vi "QuadRotor_Monitoring_WithGoogleMap.vi"() -> ()   [LabVIEW 2015]
uses:
  <vilib>/Instr/_visa.llb/VISA Set IO Buffer Mask.ctl
  <vilib>/Instr/_visa.llb/VISA Configure Serial Port (Instr).vi
panel:
  in  "Lontitude_Home":dbl=100.110974 format="%#.6g"
  in  "Latitude_Home":dbl=20.029151 format="%#.6g"
  out "URL":string="http://maps.google.com/staticmap?center=51.406200,-1.307000&zoom=18&size=570x350&maptype=hybrid&markers=51.406200,-1.307000,midpurplea&key=&path=rgb:0xFF1000,weight:5|51.406200,-1.307000|51.406200,-1.307000"
  in  "Zoom":sgl=17.0 format="%#.1g"
  in  "Y":dbl=1000.0
  in  "X":dbl=350.0
  in  "Map Format":string(combo)="hybrid"
  in  "color":string(combo)="orange"
  in  "character":string="Q"
  in  "Path Collor":u32(colorbox)=16715776
  in  "Weight":i32=5
  in  "Show Path?":bool=TRUE
  in  "Home Char":string="H"
  in  "Color":string(combo)="blue"
  in  "?":refnum<k7>(container)
  out "Target_LON":ext format="%#.7f"
  out "Target_LAT":ext format="%#.7f"
  in  "Lontitude_W3":i32=1005738310
  in  "Latitude_W3":i32=139458720
  in  "Lontitude_W2":i32=1005738310
  in  "Latitude_W2":i32=139458720
  in  "Lontitude_W1":i32=1005738310
  in  "Latitude_W1":i32=139458720
  in  "Lon_home":i32=1005748870
  in  "Lat_home":i32=139456050
  out "(GPS_numSat)":u16
  out "return count 2":u32
  out "Roob":i32
  out "Altitude_(Auto)":ext format="%#_3g"
  in  "Set_Altitude_(Auto)":dbl=2.5
  out "string":string
  out "Mode":ext format="%.2f"
  out "Altitude":dbl(slide) scale=0.0..20.0
  out "Altitude":ext format="%.2f"
  out "Yaw":dbl(knob) scale=-180.0..180.0
  out "Pitch":dbl(knob) scale=-90.0..90.0
  out "Roll":dbl(knob) scale=-90.0..90.0
  in  "Write to Quad":bool
  out "Header_58":u8
  out "GPS_Longtitude":ext format="%#.7f"
  out "Pitch":ext format="%.2f"
  out "Yaw":ext format="%.2f"
  out "GPS_Latitude":ext format="%#.7f"
  out "Roll":ext format="%.2f"
  out "return count":u32
  in  "stop":bool
  in  "VISA Serial Data":refnum<visa-resource-name>
  # "Development Autonomous Quad-Rotor Flight Controller for Medical Delivery"
  # "Home Position"
  # "9 Point"
  # "10 Point"
  # "QuadRotor Position"
  # "Data Write to Autonomous Quad Rotor (LAT 9 Point), (LON 10 Point)"
  # "Ex  13.8591411 = 138591411 , 100.5231704 = 1005231704 Using in integer  I32"
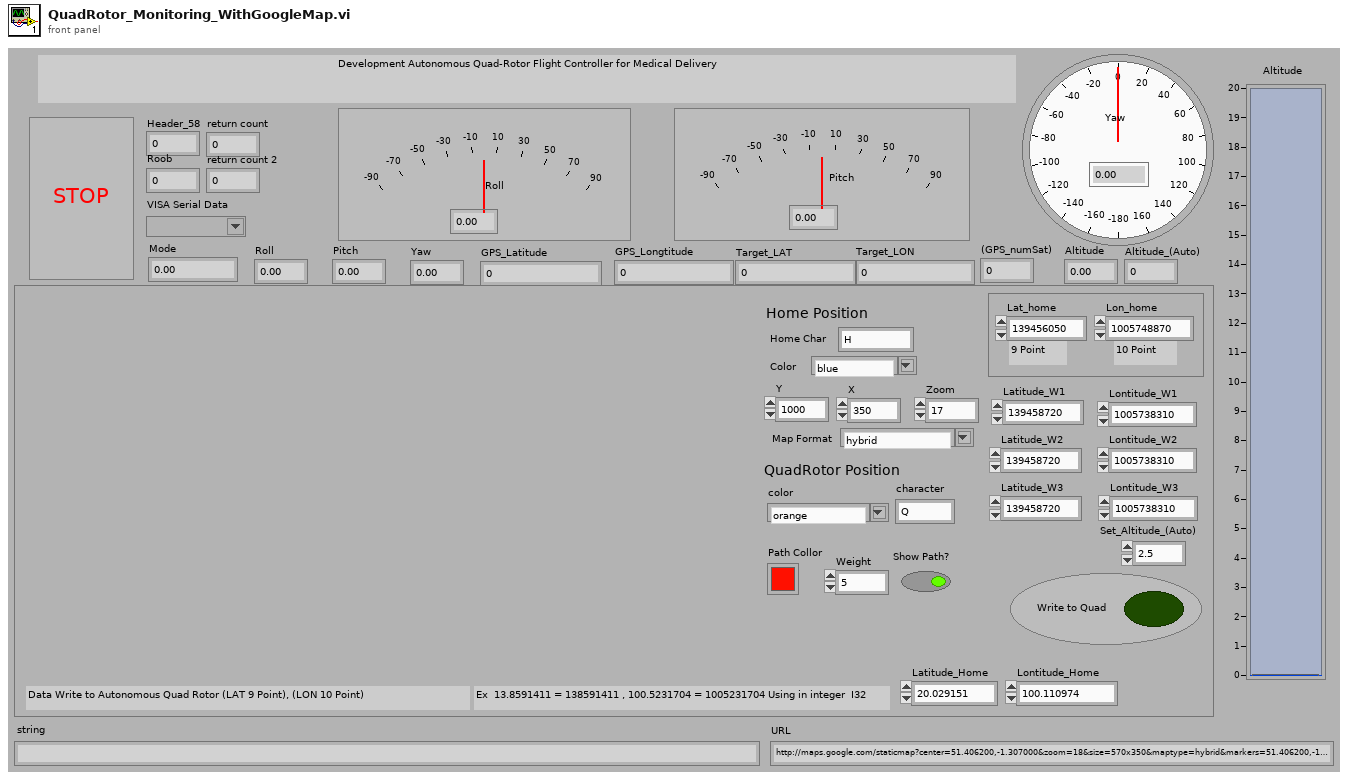
[diagram p1: front panel]
types:
  T1 = typedef "VISA Set IO Buffer Mask.ctl" = u16
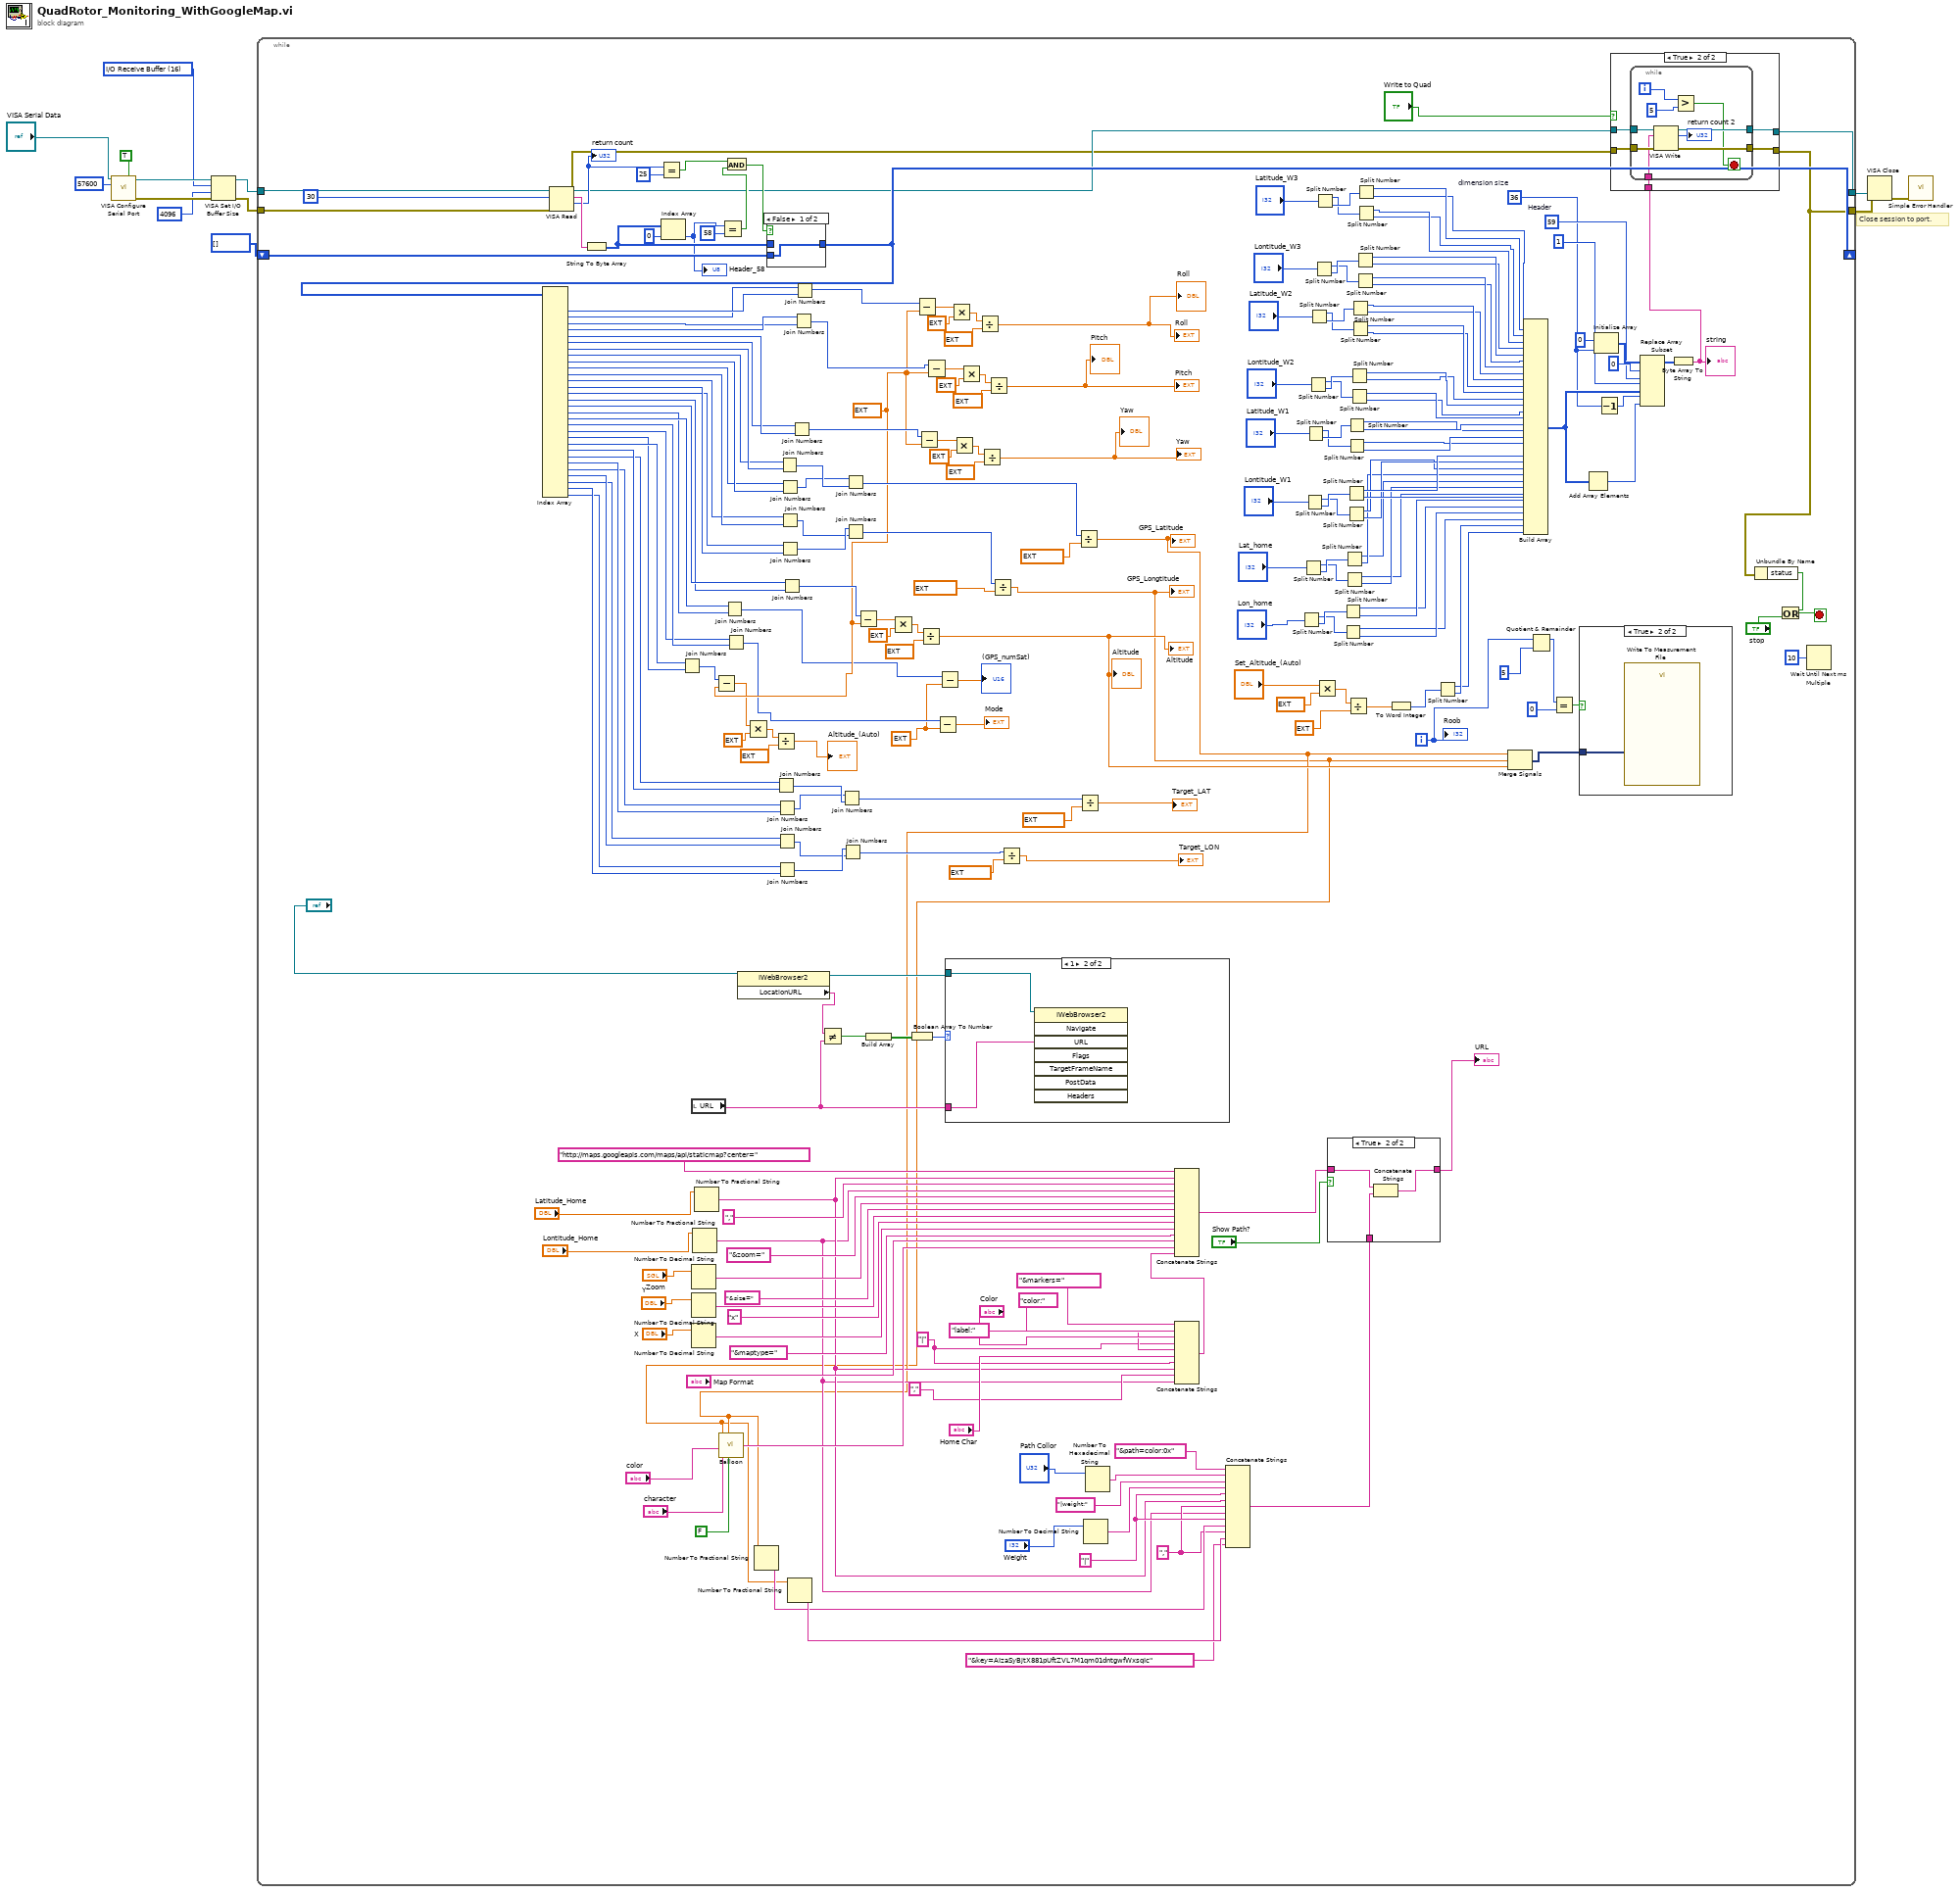
[diagram p0: block diagram]
diagram:
  w10 = T1 16 items=["I/O Receive Buffer"=16, "I/O Transmit Buffer"=32, "I/O Receive and Transmit Buffer"=48] ("Mask")
  # "Close session to port."
  n1 = call-poly "VISA Configure Serial Port"("VISA resource name"="VISA Serial Data", "Enable Termination\nChar (T)"=TRUE ("Enable Termination\nChar (T)"), "baud rate (9600)"=u32 57600) -> ("VISA resource name out"=w12:refnum<visa-resource-name>, "error out"=w11:errorcluster)  [unwired: 7 in, 4 out]
  n2 = VISA Set I/O Buffer Size(VISA resource name=w12, mask (16)=w10, size (4096)=u32 4096, error in (no error)=w11) -> (VISA resource name out=w8:refnum<visa-resource-name>, error out=w6:errorcluster)
  n3 = while {
    tunnel: [w211] -> w7
    tunnel: w8 -> [w252]
    tunnel: [w210] -> w5
    tunnel: w6 -> [w251]
    shift-right: [w221] -> _
    shift-left: u8[] [] ("unsigned byte array") -> [w222]
    i -> [w71]
    stop <- w255 stop-if-true
    w24 = "|"
    w30 = "," ("string")
    w31 = "|"
    w129 = 36  # dimension size
    w178 = u8 59  # Header
    w123 = ext 255.0 ("y")
    w139 = ext 32767.0 ("y")
    n4 = VISA Read(VISA resource name=w252, byte count=u32 30, error in (no error)=w251) -> (VISA resource name out=w213:refnum<visa-resource-name>, read buffer=w225:string, return count=w218:u32, error out=w212:errorcluster)
    "return count" <- w218
    n5 = String To Byte Array(string=w225) -> (unsigned byte array=w223:u8[])
    n6 = Equal?(x=w218, y=u32 25) -> (x = y?=w216:bool)
    n7 = Index Array(array=w223, index=0) -> (element=w215:u8)
    "Header_58" <- w215
    n8 = local read "URL"() -> (w60:string)
    n9 = Number To Decimal String(number="Zoom") -> (decimal integer string=w55:string)  [unwired: 1 in]
    n10 = Number To Decimal String(number="Y") -> (decimal integer string=w51:string)  [unwired: 1 in]
    n11 = Number To Decimal String(number="X") -> (decimal integer string=w49:string)  [unwired: 1 in]
    n12 = Number To Fractional String(number="Lontitude_Home") -> (F-format string=w21:string)  [unwired: 3 in]
    n13 = Number To Fractional String(number="Latitude_Home") -> (F-format string=w22:string)  [unwired: 3 in]
    n14 = Equal?(x=w215, y=u8 58) -> (x = y?=w220:bool)
    n15 = And(x=w216, y=w220) -> (x .and. y?=w219:bool)
    n16 = property class="IWebBrowser2"(reference="?") -> (reference out=w65:refnum<k7>, "LocationURL"=w63:string)  [unwired: 1 in, 1 out]
    n17 = case shown="False" w219 {
      tunnel: w223 -> [_ w280]
      tunnel: [w279 w280] -> w221
      tunnel: w222 -> [w279 _]
      frame False {
      }
      frame True {
      }
    }
    n18 = Index Array(array=w221) -> (element #2=w245:u8, element #3=w244:u8, element #4=w242:u8, element #5=w243:u8, element #6=w249:u8, element #7=w248:u8, element #8=w247:u8, element #9=w246:u8, element #10=w206:u8, element #11=w205:u8, element #12=w202:u8, element #13=w201:u8, element #14=w200:u8, element #15=w199:u8, element #16=w189:u8, element #17=w195:u8, element #18=w187:u8, element #19=w188:u8, element #20=w186:u8, element #21=w185:u8, element #22=w141:u8, element #23=w142:u8, element #24=w79:u8, element #25=w78:u8, element #26=w77:u8, element #27=w76:u8, element #28=w75:u8, element #29=w74:u8, element #30=w73:u8, element #31=w72:u8)  [unwired: 31 in, 1 out]
    n19 = Join Numbers(hi=w142, lo=w141) -> ((hi.lo)=w140:u16)
    n20 = Subtract(x=w140, y=w139) -> (x-y=w135:ext)
    n21 = Join Numbers(hi=w188, lo=w187) -> ((hi.lo)=w122:u16)
    n22 = Join Numbers(hi=w185, lo=w186) -> ((hi.lo)=w126:u16)
    n23 = Multiply(x=w135, y=ext 100.0) -> (x*y=w137:ext)
    n24 = Divide(x=w137, y=ext 32767.0) -> (x/y=→"Altitude_(Auto)":ext)
    n25 = Join Numbers(hi=w78, lo=w79) -> ((hi.lo)=w82:u16)
    n26 = Join Numbers(hi=w76, lo=w77) -> ((hi.lo)=w81:u16)
    n27 = Join Numbers(hi=w74, lo=w75) -> ((hi.lo)=w83:u16)
    n28 = Join Numbers(hi=w72, lo=w73) -> ((hi.lo)=w84:u16)
    n29 = Join Numbers(hi=w246, lo=w247) -> ((hi.lo)=w204:u16)
    n30 = Join Numbers(hi=w205, lo=w206) -> ((hi.lo)=w203:u16)
    n31 = Join Numbers(hi=w201, lo=w202) -> ((hi.lo)=w183:u16)
    n32 = Join Numbers(hi=w199, lo=w200) -> ((hi.lo)=w184:u16)
    n33 = Join Numbers(hi=w195, lo=w189) -> ((hi.lo)=w190:u16)
    n34 = Join Numbers(hi=w248, lo=w249) -> ((hi.lo)=w231:u16)
    n35 = Join Numbers(hi=w243, lo=w242) -> ((hi.lo)=w226:u16)
    n36 = Join Numbers(hi=w244, lo=w245) -> ((hi.lo)=w240:u16)
    n37 = Not Equal?(x=w63, y=w60) -> (x != y?=w64:bool)
    n38 = Join Numbers(hi=w81, lo=w82) -> ((hi.lo)=w80:u32)
    n39 = Join Numbers(hi=w84, lo=w83) -> ((hi.lo)=w86:u32)
    n40 = Join Numbers(hi=w203, lo=w204) -> ((hi.lo)=w208:u32)
    n41 = Join Numbers(hi=w184, lo=w183) -> ((hi.lo)=w198:u32)
    n42 = Subtract(x=w190, y=w139) -> (x-y=w194:ext)
    n43 = Build Array(w64) -> (w62:bool[])
    n44 = Multiply(x=w194, y=ext 100.0) -> (x*y=w192:ext)
    n45 = Boolean Array To Number(Boolean array=w62) -> (number=w61:u32)
    n46 = Subtract(x=w240, y=w139) -> (x-y=w239:ext)
    n47 = Subtract(x=w231, y=w139) -> (x-y=w235:ext)
    n48 = Divide(x=w192, y=ext 32767.0) -> (x/y=w121:ext)
    "Altitude" <- w121
    "Altitude" <- w121
    n49 = Subtract(x=w226, y=w139) -> (x-y=w230:ext)
    n50 = Subtract(x=w126, y=w123) -> (x-y=→"Mode":ext)
    n51 = Subtract(x=w122, y=w123) -> (x-y=→"(GPS_numSat)":ext)
    n52 = case shown="1" w61 {
      tunnel: w60 -> [_ w261]
      tunnel: w65 -> [_ w260]
      frame 0, Default {
      }
      frame 1 {
        n53 = invoke class="IWebBrowser2" method="Navigate"(reference=w260, "URL"=w261) -> ()  [unwired: 6 in, 8 out]
      }
    }
    n54 = Multiply(x=w239, y=ext 180.0) -> (x*y=w237:ext)
    n55 = Multiply(x=w235, y=ext 180.0) -> (x*y=w233:ext)
    n56 = Multiply(x=w230, y=ext 180.0) -> (x*y=w228:ext)
    n57 = Divide(x=w237, y=ext 32767.0) -> (x/y=→"Roll" →"Roll":ext)
    n58 = Divide(x=w233, y=ext 32767.0) -> (x/y=→"Yaw" →"Yaw":ext)
    n59 = Divide(x=w228, y=ext 32767.0) -> (x/y=→"Pitch" →"Pitch":ext)
    n60 = Divide(x=w198, y=ext 10000000.0) -> (x/y=w14:ext)
    "GPS_Longtitude" <- w14
    n61 = Number To Fractional String(number=w14) -> (F-format string=w33:string)  [unwired: 3 in]
    n62 = Divide(x=w86, y=ext 10000000.0) -> (x/y=→"Target_LON":ext)
    n63 = Divide(x=w208, y=ext 10000000.0) -> (x/y=w15:ext)
    "GPS_Latitude" <- w15
    n64 = call "Balloon.vi"("One more?"=FALSE, "Latitude"=w15, "character"="character", "color"="color", "Longitude"=w14) -> ("Balloon"=w46:string)  [unwired: 1 in]
    n65 = Number To Fractional String(number=w15) -> (F-format string=w32:string)  [unwired: 3 in]
    n66 = Divide(x=w80, y=ext 10000000.0) -> (x/y=→"Target_LAT":ext)
    n67 = Number To Decimal String(number="Weight") -> (decimal integer string=w37:string)  [unwired: 1 in]
    n68 = Number To Hexadecimal String(2:"Path Collor") -> (0:w40:string)  [unwired: 1 in]
    n69 = Concatenate Strings("&markers=", "color:", "Color", w24, "label:", "Home Char", w24, w22, ",", w21) -> (w20:string)
    n70 = Concatenate Strings("http://maps.googleapis.com/maps/api/staticmap?center=" ("URL"), w22, "," ("string"), w21, "&zoom=", w55, "&size=", w51, "x", w49, "&maptype=", "Map Format", w46, w20) -> (w34:string)
    n71 = Concatenate Strings("&path=color:0x" ("string"), w40, "|weight:", w37, w31, w22, w30, w21, w31, w32, w30, w33, "&key=AIzaSyBjtX881pUftZVL7M1qm01dntgwfWxsqIc" ("string")) -> (w19:string)
    n72 = Split Number(x="Lon_home") -> (hi(x)=w171:u16, lo(x)=w172:u16)
    n73 = Split Number(x="Lat_home") -> (hi(x)=w173:u16, lo(x)=w174:u16)
    n74 = Split Number(x="Lontitude_W1") -> (hi(x)=w175:u16, lo(x)=w176:u16)
    n75 = Split Number(x="Latitude_W1") -> (hi(x)=w153:u16, lo(x)=w154:u16)
    n76 = Split Number(x="Lontitude_W2") -> (hi(x)=w114:u16, lo(x)=w115:u16)
    n77 = Split Number(x="Latitude_W2") -> (hi(x)=w112:u16, lo(x)=w113:u16)
    n78 = Split Number(x="Lontitude_W3") -> (hi(x)=w108:u16, lo(x)=w109:u16)
    n79 = Split Number(x="Latitude_W3") -> (hi(x)=w106:u16, lo(x)=w107:u16)
    n80 = Multiply(x="Set_Altitude_(Auto)", y=ext 32767.0) -> (x*y=w145:ext)
    n81 = case shown="True" "Show Path?" {
      tunnel: w19 -> [_ w259]
      tunnel: [w256 w258] -> w35
      tunnel: w34 -> [w256 w257]
      frame False {
      }
      frame True {
        n82 = Concatenate Strings(w257, w259) -> (w258:string)
      }
    }
    "URL" <- w35
    n83 = Split Number(x=w172) -> (hi(x)=w157:u8, lo(x)=w158:u8)
    n84 = Split Number(x=w171) -> (hi(x)=w155:u8, lo(x)=w156:u8)
    n85 = Split Number(x=w174) -> (hi(x)=w161:u8, lo(x)=w162:u8)
    n86 = Split Number(x=w173) -> (hi(x)=w159:u8, lo(x)=w160:u8)
    n87 = Split Number(x=w176) -> (hi(x)=w165:u8, lo(x)=w166:u8)
    n88 = Split Number(x=w175) -> (hi(x)=w163:u8, lo(x)=w164:u8)
    n89 = Split Number(x=w154) -> (hi(x)=w169:u8, lo(x)=w170:u8)
    n90 = Split Number(x=w153) -> (hi(x)=w167:u8, lo(x)=w168:u8)
    n91 = Divide(x=w145, y=ext 100.0) -> (x/y=w143:ext)
    n92 = Split Number(x=w115) -> (hi(x)=w101:u8, lo(x)=w100:u8)
    n93 = Split Number(x=w114) -> (hi(x)=w103:u8, lo(x)=w102:u8)
    n94 = Split Number(x=w113) -> (hi(x)=w97:u8, lo(x)=w96:u8)
    n95 = Split Number(x=w112) -> (hi(x)=w99:u8, lo(x)=w98:u8)
    n96 = Split Number(x=w109) -> (hi(x)=w93:u8, lo(x)=w92:u8)
    n97 = Split Number(x=w108) -> (hi(x)=w95:u8, lo(x)=w94:u8)
    n98 = Split Number(x=w107) -> (hi(x)=w89:u8, lo(x)=w88:u8)
    n99 = Split Number(x=w106) -> (hi(x)=w91:u8, lo(x)=w90:u8)
    n100 = To Word Integer(number=w143) -> (16bit integer=w146:i16)
    n101 = Split Number(x=w146) -> (hi(x)=w147:u8, lo(x)=w148:u8)
    n102 = Merge Signals(w15, w14, w121) -> (w120:dynamicdata)
    n103 = Build Array(w88, w89, w90, w91, w92, w93, w94, w95, w96, w97, w98, w99, w100, w101, w102, w103, w170, w169, w168, w167, w166, w165, w164, w163, w162, w161, w160, w159, w158, w157, w156, w155, w148, w147) -> (w132:u8[])
    n104 = Quotient & Remainder(x=w71, y=u32 5) -> (x-y*floor(x/y)=w116:u32)  [unwired: 1 out]
    n105 = Equal?(x=w116, y=u32 0) -> (x = y?=w118:bool)
    n106 = case shown="True" w118 {
      tunnel: w120 -> [_ w262]
      frame False {
      }
      frame True {
        n107 = call "Write To Measurement File"("Signals"=w262) -> ()  [unwired: 16 in, 3 out]
      }
    }
    n108 = Add Array Elements(numeric array=w132) -> (sum=w131:u8)
    n109 = Initialize Array(u8 0, w129) -> (w182:u8[])
    n110 = Decrement(x=w129) -> (x-1=w130:i32)
    n111 = Replace Array Subset(array=w182, new element #1=w178, index #1=0 ("index"), new element #2=w132, index #2=1 ("index"), new element #3=w131, index #3=w130) -> (w177:u8[])
    n112 = Byte Array To String(unsigned byte array=w177) -> (string=w152:string)
    "string" <- w152
    n113 = case shown="True" "Write to Quad" {
      tunnel: w213 -> [w263 w269]
      tunnel: w212 -> [w264 w266]
      tunnel: [w263 w268] -> w211
      tunnel: [w264 w267] -> w210
      tunnel: w152 -> [_ w265]
      frame False {
      }
      frame True {
        n114 = while {
          tunnel: w269 -> [w278]
          tunnel: [w277] -> w268
          tunnel: [w276] -> w267
          tunnel: w266 -> [w275]
          tunnel: w265 -> [w274]
          i -> [w272]
          stop <- w270 stop-if-true
          n115 = VISA Write(VISA resource name=w278, write buffer=w274, error in (no error)=w275) -> (VISA resource name out=w277:refnum<visa-resource-name>, return count=→"return count 2":u32, error out=w276:errorcluster)
          n116 = Greater?(x=w272, y=5) -> (0:w270:bool)
        }
      }
    }
    n117 = Unbundle By Name(w210) -> ("status"=w253:bool)
    n118 = Or(x=w253, y="stop") -> (x .or. y?=w255:bool)
    n119 = Wait Until Next ms Multiple(millisecond multiple=u32 10) -> ()  [unwired: 1 out]
    "Roob" <- w71
  }
  n120 = VISA Close(VISA resource name=w7, error in (no error)=w5) -> (error out=w9:errorcluster)
  n121 = call <vilib>:"Simple Error Handler.vi"("error in (no error)"=w9) -> ()  [unwired: 1 in, 8 out]
